vi "repeat_waveform.vi"(8 "waveform repetitions":i32, 11 "signal in":waveform(dbl)) -> (0 "waveform length":i32, 3 "signal out":waveform(dbl))   [LabVIEW 2019]
panel:
  out "signal out":waveform(dbl)(graph)
  out "signal in":waveform(dbl)(graph)
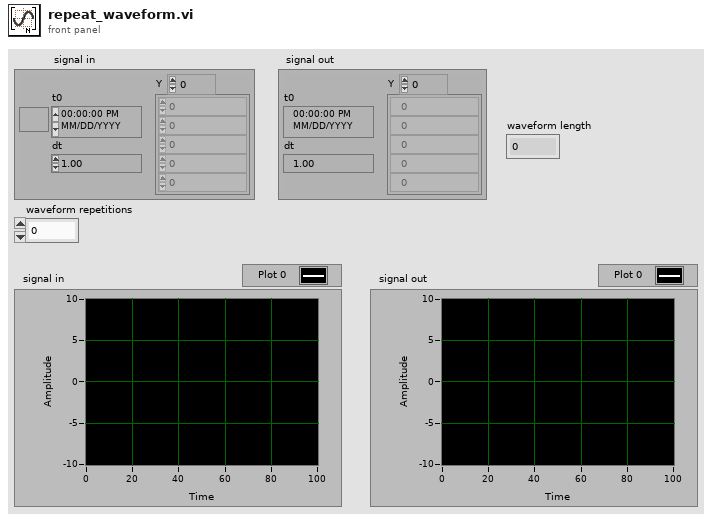
[diagram p1: front panel]
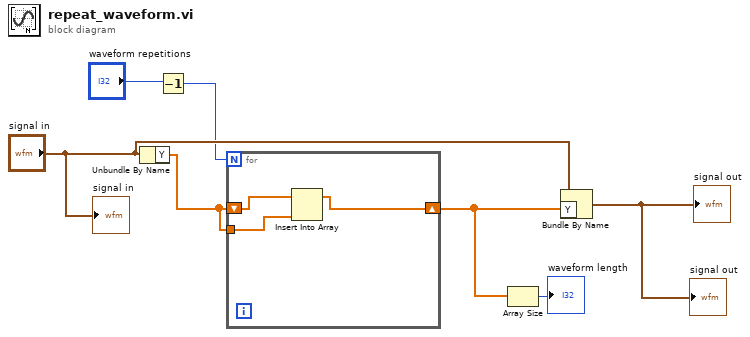
[diagram p0: block diagram]
diagram:
  n1 = Unbundle By Name("signal in") -> ("Y"=w7:dbl[])
  n2 = Decrement(x="waveform repetitions") -> (x-1=w1:i32)
  n3 = for {
    N: w1 -> [_]
    shift-right: [w8] -> w4
    shift-left: w7 -> [w10]
    tunnel: w7 -> [w9]
    n4 = Insert Into Array(array=w10, new element=w9) -> (w8:dbl[])  [unwired: 1 in]
  }
  n5 = Array Size(array=w4) -> (size(s)=→"waveform length":i32)
  n6 = Bundle By Name(cluster="signal in", "Y"=w4) -> (→"signal out" →"signal out":waveform(dbl))
  "signal in" <- "signal in"
